vi "Decode Plugin Tree Tag.vi"(8 "error in (no error)":errorcluster, 11 "Tag":string) -> (0 "error out":errorcluster, 3 "Plugin Tree Tag":T1)   [LabVIEW 2018]
uses:
  Controls/Plugin Tree Tag.ctl
  Controls/Plugins Tree Item Type.ctl
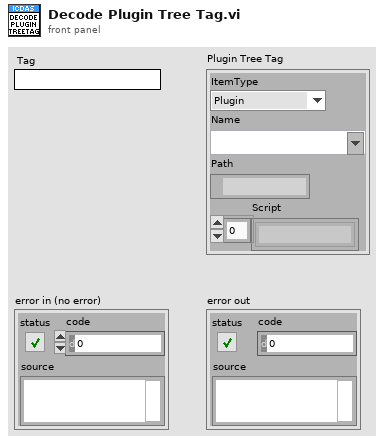
[diagram p1: front panel]
types:
  T1 = typedef "Plugin Tree Tag.ctl" = cluster{"ItemType":T2, "Name":string, "Path":path, "Script":string[]}
  T2 = typedef "Plugins Tree Item Type.ctl" = enum16{"Plugin", "Instrument", "INI File", "INI Script"}
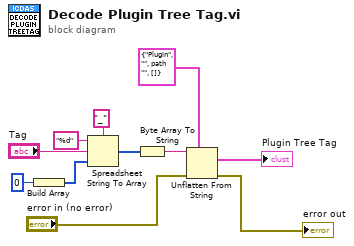
[diagram p0: block diagram]
diagram:
  n1 = Build Array(u8 0 ("HygroID")) -> (w6:u8[])
  n2 = Spreadsheet String To Array(delimiter (Tab)="_", format string="%d", spreadsheet string="Tag", array type (2D Dbl)=w6) -> (array=w7:u8[])
  n3 = Byte Array To String(unsigned byte array=w7) -> (string=w5:string)
  n4 = Unflatten From String(type=T1 {"ItemType"=enum."Plugin", "Name"="", "Path"=path "", "Script"=[]} ("Test Manager Tree Tag"), binary string=w5, error in (no error)="error in (no error)") -> (value=→"Plugin Tree Tag":T1, error out=→"error out":errorcluster)  [unwired: 2 in, 1 out]
